vi "SafeTip.vi"() -> ()   [LabVIEW 2016]
uses:
  controls/Enum.ctl
  Course Project/support/Message Queue/Message Cluster.ctl
  <vilib>/Utility/error.llb/Error Cluster From Error Code.vi
  <vilib>/rvi/errors/niLvFpgaAdjustHostInterfaceError.vi
  <vilib>/rvi/interface/nirviReadWriteControl/nirviReadWriteControl.xnode
  controls/FPGAVIreferenceTypeDefScanEngine.ctl
  FPGA Bitfiles/qnmController797_usbRIO_controllerFPGAmu.lvbitx
  Course Project/support/Message Queue/Message Queue.lvlib
  NiFpgaLv.dll
panel:
  out "SafeTipParametersIn":T1 {"SafeTipSignal" items=["AI0", "AI1", "AI2", "AI3", "AI4", "AI5", "AI6", "AI7"]}
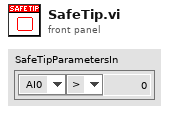
[diagram p1: front panel]
types:
  T1 = cluster{"SafeTipValue":dbl, ">/<":enum16{">", "<"}, "SafeTipSignal":u16}
  T2 = typedef "Enum.ctl" = enum16{"Init", "Read", "Write"}
  T3 = typedef "FPGAVIreferenceTypeDefScanEngine.ctl" = refnum<k20>
  T4 = typedef "Message Queue.lvlib/Message Cluster.ctl" = cluster{"Message":string, "Données de message":variant}
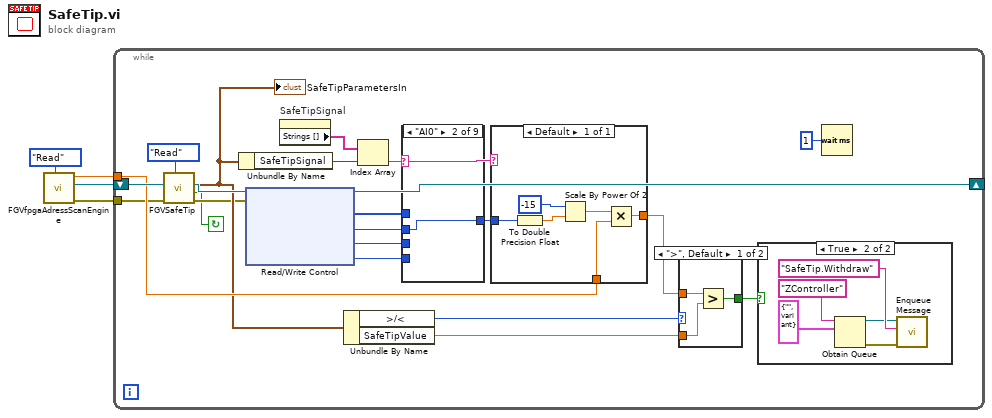
[diagram p0: block diagram]
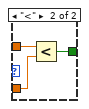
[diagram p3: hidden frame]
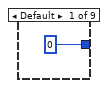
[diagram p4: hidden frame]
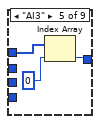
[diagram p7: hidden frame]
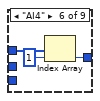
[diagram p8: hidden frame]
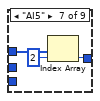
[diagram p9: hidden frame]
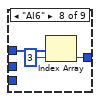
[diagram p10: hidden frame]
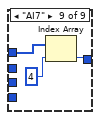
[diagram p11: hidden frame]
diagram:
  n1 = call "FGVfpgaAdressScanEngine.vi"("Enum"=Enum."Read") -> ("error out"=w3:errorcluster, "FPGA.SEout"=w2:T3, "voltageRange(+/-)Out"=w1:dbl)  [unwired: 6 in, 2 out]
  n2 = while {
    tunnel: w3 -> [w10]
    tunnel: w1 -> [w16]
    shift-right: [w5] -> _
    shift-left: w2 -> [w17]
    stop <- w8 continue-if-true
    n3 = call "FGVSafeTip.vi"("Enum"=Enum."Read", "error in"=w10) -> ("error out"=w9:errorcluster, "SafeTipOn?"=w8:bool, "SafeTipParametersOut"=w14:T1)  [unwired: 7 in]
    "SafeTipParametersIn" <- w14
    n4 = Unbundle By Name(w14) -> ("SafeTipSignal"=w18:u16)
    n5 = xnode "Read/Write Control"("FPGA VI Reference In"=w17, "error in"=w9) -> ("FPGA VI Reference Out"=w5:T3, "aio.o.inputs"=w24:i16[], "aio.s.slowVertical"=w23:i16, "aio.s.slowHoriz"=w22:i16, "aio.s.sum"=w21:i16)  [unwired: 1 out]
    n6 = property on="SafeTipSignal" class="Ring (strict)"() -> ("Strings []"=w15:string[])  [unwired: 2 in, 2 out]
    n7 = Unbundle By Name(w14) -> (">/<"=w13:enum16{">", "<"}, "SafeTipValue"=w11:dbl)
    n8 = Index Array(array=w15, index=w18) -> (element=w19:string)
    n9 = case shown="\"AI0\"" w19 {
      tunnel: w24 -> [_ _ _ _ w49 w50 w53 w56 w60]
      tunnel: w23 -> [_ w44 _ _ _ _ _ _ _]
      tunnel: w22 -> [_ _ w45 _ _ _ _ _ _]
      tunnel: w21 -> [_ _ _ w46 _ _ _ _ _]
      tunnel: [0 ("aio.s.slowVertical") w44 w45 w46 w48 w51 w54 w57 w59] -> w20
      frame Default {
      }
      frame "AI0" {
      }
      frame "AI1" {
      }
      frame "AI2" {
      }
      frame "AI3" {
        n10 = Index Array(array=w49, index=0) -> (element=w48:i16)
      }
      frame "AI4" {
        n11 = Index Array(array=w50, index=1) -> (element=w51:i16)
      }
      frame "AI5" {
        n12 = Index Array(array=w53, index=2) -> (element=w54:i16)
      }
      frame "AI6" {
        n13 = Index Array(array=w56, index=3) -> (element=w57:i16)
      }
      frame "AI7" {
        n14 = Index Array(array=w60, index=4) -> (element=w59:i16)
      }
    }
    n15 = case shown="Default" w19 {
      tunnel: w20 -> [w40]
      tunnel: [w38] -> w12
      tunnel: w16 -> [w37]
      frame Default {
        n16 = To Double Precision Float(number=w40) -> (double precision float=w42:dbl)
        n17 = Scale By Power Of 2(n=i16 -15, x=w42) -> (x*2^n=w39:dbl)
        n18 = Multiply(x=w39, y=w37) -> (x*y=w38:dbl)
      }
    }
    n19 = case shown="\">\", Default" w13 {
      tunnel: w12 -> [w33 w36]
      tunnel: w11 -> [w32 w35]
      tunnel: [w31 w34] -> w7
      frame ">", Default {
        n20 = Greater?(x=w33, y=w32) -> (0:w31:bool)
      }
      frame "<" {
        n21 = Less?(x=w36, y=w35) -> (x < y?=w34:bool)
      }
    }
    n22 = case shown="True" w7 {
      frame False {
      }
      frame True {
        n23 = Obtain Queue(name (unnamed)="ZController" ("QueueName"), element data type=T4 {"Message"="", "Données de message"=variant} ("Cluster Message")) -> (queue out=w26:refnum<queue>, error out=w28:errorcluster)  [unwired: 3 in, 1 out]
        n24 = call "Enqueue Message.vi"("error in"=w28, "Message"="SafeTip.Withdraw", "Queue"=w26) -> ()  [unwired: 7 in, 2 out]
      }
    }
    n25 = Wait (ms)(milliseconds to wait=u32 1) -> ()  [unwired: 1 out]
  }
